vi "Create from Session.vi"(8 "Error In":errorcluster, 10 "Port":i32, 11 "Session":refnum<class "Session.lvclass">) -> (0 "Error Out":errorcluster, 3 "Listener":refnum<class "Listener.lvclass">)   [LabVIEW 2018, in "Toolkit.lvlib" / "Listener.lvclass"]
uses:
  Listener.lvclass
  Session/Session.lvclass
  Session/Session.lvclass/Session.ctl
  SSH/SSH.lvclass/SSH.ctl
  Listener.lvclass/Listener.ctl
  Toolkit.lvlib
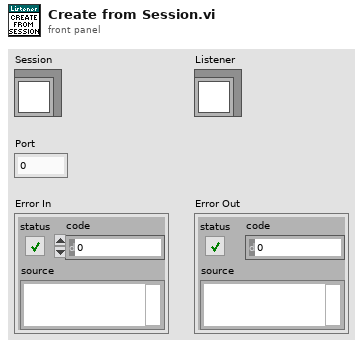
[diagram p1: front panel]
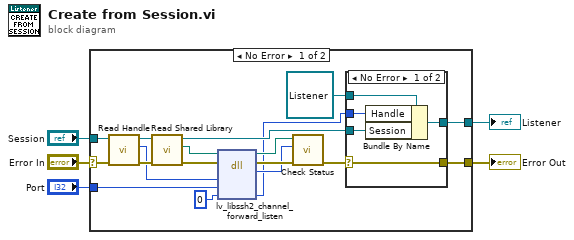
[diagram p0: block diagram]
diagram:
  n1 = case shown="No Error" "Error In" {
    selector: "Error In" -> [w16 w31]
    tunnel: [w18 w31] -> w4
    tunnel: [w23 _] -> w1
    tunnel: "Session" -> [w17 _]
    tunnel: "Port" -> [w7 _]
    frame No Error {
      n2 = call "Read Handle.vi"("Error In"=w16, "Session In"=w17) -> ("Erorr Out"=w14:errorcluster, "Handle"=w9:u64, "Session Out"=w15:refnum<class "Session.lvclass">)  [unwired: 7 in]
      n3 = call "Read Shared Library.vi"("Error In"=w14, "Session In"=w15) -> ("Erorr Out"=w10:errorcluster, "libssh2lv Shared Library"=w11:path, "Session Out"=w12:refnum<class "Session.lvclass">)  [unwired: 7 in]
      n4 = dll-call lib="lv-libssh2.*" fn="lv_libssh2_channel_forward_listen"(path in=w11, error in=w10, "session"=w9, "port"=w7, "handle"=u64 0) -> (path out=w21:path, error out=w22:errorcluster, "status"=w20:i32, "handle"=w8:u64)  [unwired: 3 in]
      n5 = call "Check Status.vi"("Error In"=w22, "Status"=w20, "lv-libssh2 Shared Library In"=w21) -> ("Error Out"=w19:errorcluster)  [unwired: 7 in, 1 out]
      n6 = case shown="No Error" w19 {
        selector: w19 -> [w27 w30]
        tunnel: [w28 w29] -> w23
        tunnel: [w27 w30] -> w18
        tunnel: w12 -> [w26 _]
        tunnel: refnum<class "Listener.lvclass"> refnum ("Toolkit.lvlib:Listener.lvclass") -> [w25 w29]
        tunnel: w8 -> [w24 _]
        frame No Error {
          n7 = Bundle By Name(cluster=w25, "Handle"=w24, "Session"=w26) -> (w28:refnum<class "Listener.lvclass">)
        }
        frame Error {
        }
      }
    }
    frame Error {
    }
  }
  "Error Out" <- w4
  "Listener" <- w1
